vi "Autonomous Independent.vi"() -> ()   [LabVIEW 2015]
doc: "This VI is called when autonomous begins, and will automatically be terminated when autonomous ends. You can carry out timed or sensor driven robot movement independently without needing to return to the caller."
uses:
  <vilib>/Rock Robotics/WPI/SafetyOutput/WPI_SafetyOutputConfigMenu.ctl
  <vilib>/Rock Robotics/WPI/Utilities/WPI_GetSetVariantRefNum.vi
  <vilib>/Rock Robotics/Network Tables/NT Read String.vi
  <vilib>/Rock Robotics/Network Tables/NT Write Numeric Array.vi
  <vilib>/Rock Robotics/Network Tables/NT Read Number.vi
  <vilib>/Rock Robotics/WPI/Ultrasonic/WPI_SonarMB1010AnalogRefNum Registry Get.vi
  navx-mxp/labview/navX Library v2/navX Library v2.lvlib
panel:
  out "Distance":dbl
  out "Numeric 2":dbl
  out "Numeric":dbl
  # "Be sure to right-click and choose Data Operations>>Make Current Value default if you want to save the array values with the VI"
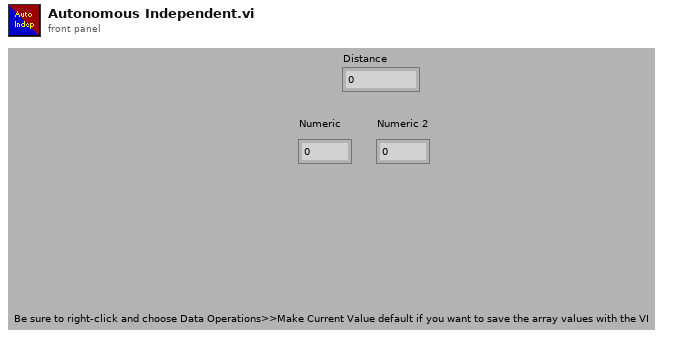
[diagram p1: front panel]
types:
  T1 = typedef "WPI_SafetyOutputConfigMenu.ctl" = enum16{"Enable", "Disable"}
  T2 = typedef "WPI_JoystickDevRef.ctl" = cluster{"Device":T3}
  T3 = typedef "WPI_JoystickDeviceEnum.ctl" = enum16{"USB 0", "USB 1", "USB 2", "USB 3", "USB 4", "USB 5"}
  T4 = typedef "WPI_RobotDriveDevRef.ctl" = cluster{"DevStatus":errorcluster, "Motors[]":T5[], "Square Inputs":bool, "Max Output":dbl}
  T5 = typedef "WPI_MotorControlDeviceRef.ctl" = cluster{"DeviceStatus":errorcluster, "Type":T6, "PWM":cluster{"PWM Channel":T7, "DeadBand":T8}, "CAN":cluster{"Device Number":u8, "Control Mode":T9, "Semaphore":T10, "Max Vout":dbl, "TalonSRX Control Mode":T11}, "Invert":bool}
  T6 = typedef "WPI_MotorControlType.ctl" = enum16{"PWM", "CAN", "CANTalonSRX"}
  T7 = typedef "FPGA_DIOPWMChannel.ctl" = enum8{"PWM 0", "PWM 1", "PWM 2", "PWM 3", "PWM 4", "PWM 5", "PWM 6", "PWM 7", "PWM 8", "PWM 9", "PWM MXP 0", "PWM MXP 1", "PWM MXP 2", "PWM MXP 3", "PWM MXP 4", "PWM MXP 5", "PWM MXP 6", "PWM MXP 7", "PWM MXP 8", "PWM MXP 9", "Invalid"}
  T8 = typedef "WPI_PWMDeadband.ctl" = cluster{"Name":string, "maxPositivePwm":i32, "minPositivePwm":i32, "centerPwm":i32, "maxNegativePwm":i32, "minNegativePwm":i32, "angularRange":u16}
  T9 = typedef "WPI_CANJaguar_ControlMode.ctl" = enum8{"Percent VBus", "Current", "Speed", "Position", "Voltage"}
  T10 = typedef "Semaphore RefNum" = refnum<k1>
  T11 = typedef "WPI_CANTalonSRX_APIControlMode.ctl" = enum8{"Percent VBus", "Speed", "Position", "Slave", "Unchanged / Invalid", "Voltage Compensation", "Current", "Motion Profile"}
  T12 = typedef "navX Library v2.lvlib/Z900_navX_DeviceTypeDef.ctl" = cluster{"Interface":cluster{"Protocol":T13, "Update Rate (4Hz-60Hz)":u8, "navX Open TypeDef":variant}, "Notify Packet":refnum<notifier>, "Loop VI Refnum":refnum<vi>, "Ready to Close Occurrence Refnum":refnum<k4>}
  T13 = typedef "navX Library v2.lvlib/Z900_navX_ProtocolTypeDef.ctl" = enum16{"SERIAL", "I2C", "SPI"}
  T14 = typedef "WPI_EncoderDevRef.ctl" = cluster{"DevStatus":errorcluster, "EncoderIndex":T15, "CounterIndex":T16, "DistancePerCount":dbl, "Decoding Type":T17}
  T15 = typedef "FPGA_EncoderIdx.ctl" = enum8{"Enc 0", "Enc 1", "Enc 2", "Enc 3", "Enc 4", "Enc 5", "Enc 6", "Enc 7", "Invalid"}
  T16 = typedef "FPGA_CounterCtrSystemIndex.ctl" = enum8{"Ctr 0", "Ctr 1", "Ctr 2", "Ctr 3", "Ctr 4", "Ctr 5", "Ctr 6", "Ctr 7", "Invalid"}
  T17 = typedef "WPI_EncoderType.ctl" = enum16{"1x", "2x", "4x"}
  T18 = typedef "WPI_SonarMB1010AnalogDeviceRef.ctl" = cluster{"AIDeviceRef":T19, "Scaling factor (V/in)":dbl, "Average Bits":u8}
  T19 = typedef "WPI_AnalogChannelDevRef.ctl" = cluster{"DevStatus":errorcluster, "Analog Channel":T20}
  T20 = typedef "FPGA_AIChannel.ctl" = enum8{"AI 0", "AI 1", "AI 2", "AI 3", "AI MXP 0", "AI MXP 1", "AI MXP 2", "AI MXP 3", "Invalid"}
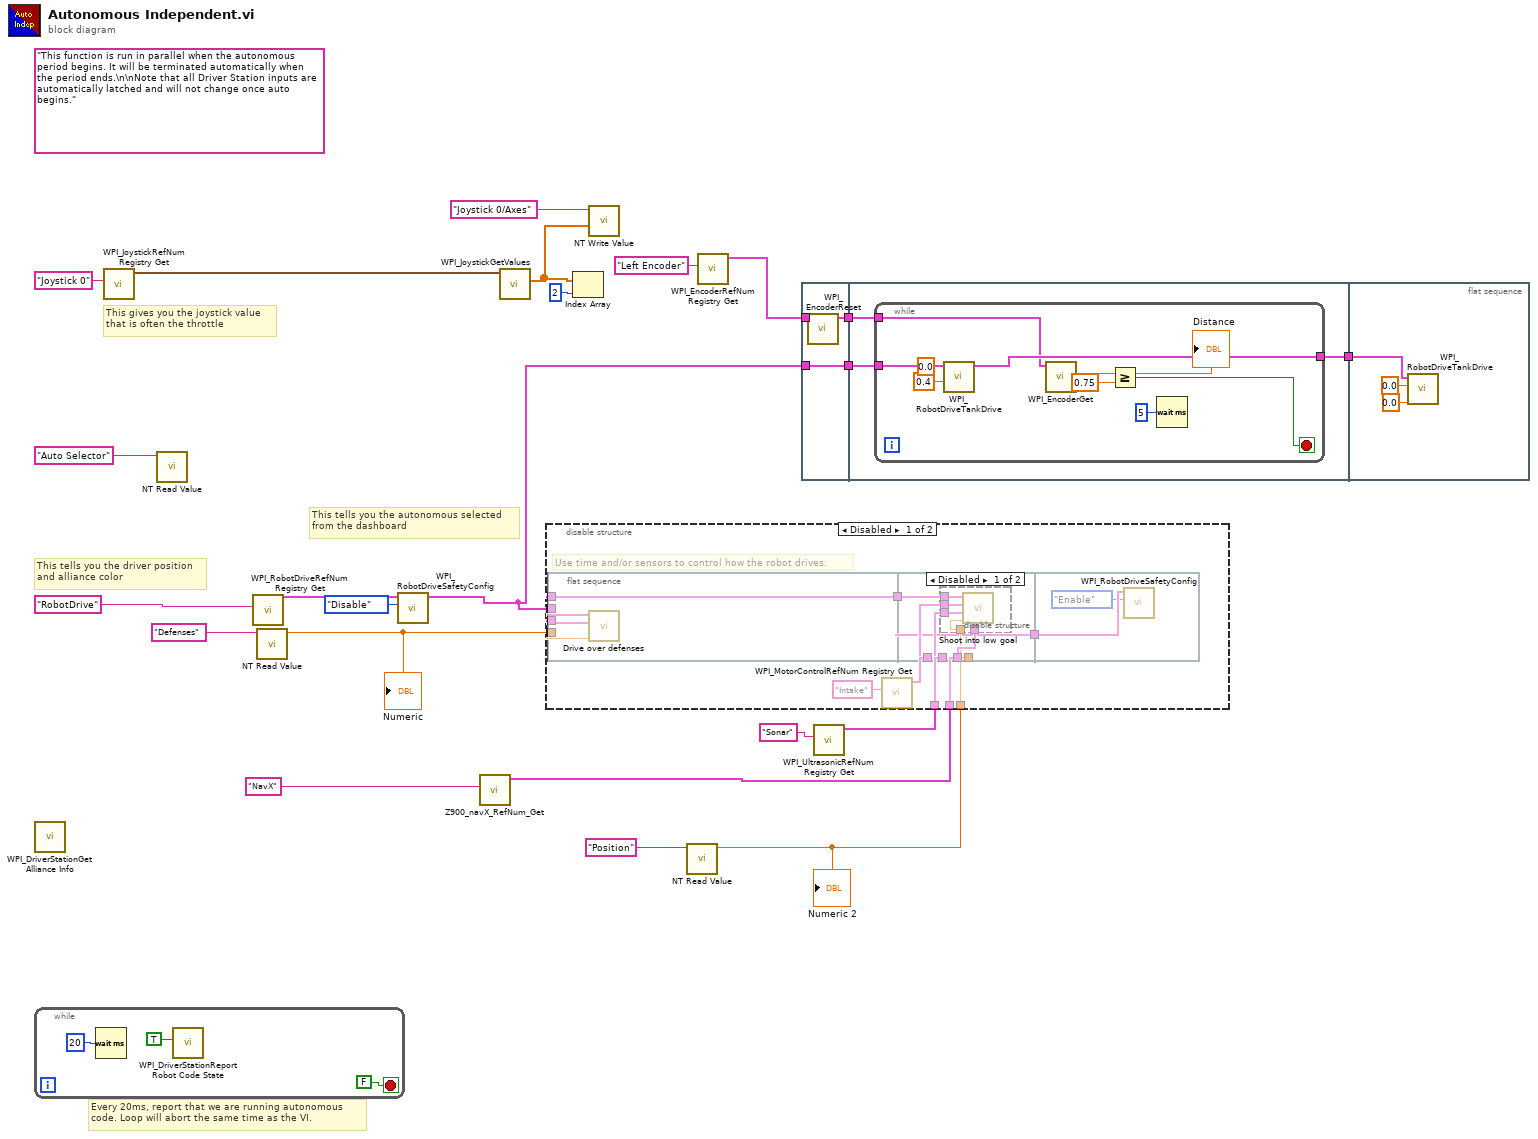
[diagram p0: block diagram]
diagram:
  (unwired) "This function is run in parallel when the autonomous period begins. It will be terminated automatically when the period ends.\n\nNote that all Driver Station inputs are automatically latched and will not change once auto begins."
  # "This tells you the autonomous selected\nfrom the dashboard"
  # "Every 20ms, report that we are running autonomous\ncode. Loop will abort the same time as the VI."
  # "This gives you the joystick value\nthat is often the throttle"
  # "This tells you the driver position\nand alliance color"
  n1 = call <vilib>:"WPI_DriverStationGet Alliance Info.vi"() -> ()  [unwired: 12 out]
  n2 = while {
    stop <- FALSE stop-if-true
    n3 = Wait (ms)(milliseconds to wait=u32 20) -> ()  [unwired: 1 out]
    n4 = call <vilib>:"WPI_DriverStationReport Robot Code State.vi"("Autonomous"=TRUE) -> ()  [unwired: 10 in, 1 out]
  }
  n5 = call <vilib>:"WPI_JoystickRefNum Registry Get.vi"("refnum name"="Joystick 0") -> ("JoystickDevRef"=w22:T2)  [unwired: 1 in, 9 out]
  n6 = call-poly <vilib>:"NT Read Value.vi"("Name"="Auto Selector") -> ()  [unwired: 9 in, 2 out]
  n7 = call <vilib>:"WPI_RobotDriveRefNum Registry Get.vi"("refnum name"="RobotDrive") -> ("RobotDriveDevRef"=w7:T4)  [unwired: 9 in, 1 out]
  n8 = call-poly <vilib>:"NT Read Value.vi"("Name"="Defenses") -> ("Numeric"=w13:dbl)  [unwired: 9 in, 1 out]
  "Numeric" <- w13
  n9 = call <vilib>:"WPI_RobotDriveSafetyConfig.vi"("mode"=WPI_SafetyOutputConfigMenu."Disable", "RobotDriveDevRef"=w7) -> ("RobotDriveDevRef"=w5:T4)  [unwired: 8 in, 1 out]
  n10 = call "Z900_navX_RefNum_Get.vi"("refnum name"="NavX") -> ("navX Device"=w9:T12)  [unwired: 9 in, 1 out]
  n11 = call <vilib>:"WPI_JoystickGetValues.vi"("JoystickDevRef"=w22) -> ("Axes"=w19:dbl[])  [unwired: 6 in, 4 out]
  n12 = Index Array(array=w19, index=2) -> ()  [unwired: 1 out]
  n13 = call-poly <vilib>:"NT Write Value.vi"("Numeric Array"=w19, "Name"="Joystick 0/Axes") -> ()  [unwired: 9 in, 1 out]
  n14 = call-poly <vilib>:"NT Read Value.vi"("Name"="Position") -> ("Numeric"=w8:dbl)  [unwired: 9 in, 1 out]
  "Numeric 2" <- w8
  n15 = call <vilib>:"WPI_EncoderRefNum Registry Get.vi"("refnum name"="Left Encoder") -> ("EncoderDevRef"=w2:T14)  [unwired: 9 in, 1 out]
  n16 = flat-sequence {
    tunnel: w5 -> [w29]
    tunnel: [w29] -> w3
    tunnel: w2 -> [w28]
    tunnel: [w27] -> w1
    tunnel: [w31] -> w4
    tunnel: w3 -> [w32]
    tunnel: w1 -> [w30]
    tunnel: w4 -> [w42]
    frame #0 {
      n17 = call <vilib>:"WPI_EncoderReset.vi"("EncoderDevRef"=w28) -> ("EncoderDevRef"=w27:T14)  [unwired: 9 in, 1 out]
    }
    frame #1 {
      n18 = while {
        tunnel: w32 -> [w41]
        tunnel: [w34] -> w31
        tunnel: w30 -> [w33]
        stop <- w36 stop-if-true
        n19 = call <vilib>:"WPI_RobotDriveTankDrive.vi"("Right axis value"=0.4, "Left axis value"=0.0, "RobotDriveDevRef"=w41) -> ("RobotDriveDevRef"=w34:T4)  [unwired: 6 in, 2 out]
        n20 = call <vilib>:"WPI_EncoderGet.vi"("EncoderDevRef"=w33) -> ("Distance"=w38:dbl)  [unwired: 5 in, 5 out]
        "Distance" <- w38
        n21 = Greater Or Equal?(x=w38, y=0.75) -> (x >= y?=w36:bool)
        n22 = Wait (ms)(milliseconds to wait=u32 5) -> ()  [unwired: 1 out]
      }
    }
    frame #2 {
      n23 = call <vilib>:"WPI_RobotDriveTankDrive.vi"("Right axis value"=0.0, "Left axis value"=0.0, "RobotDriveDevRef"=w42) -> ()  [unwired: 6 in, 3 out]
    }
  }
  n24 = call-poly <vilib>:"WPI_UltrasonicRefNum Registry Get.vi"("refnum name"="Sonar") -> ("SonarMB1010AnalogDevRef"=w10:T18)  [unwired: 9 in, 1 out]
  n25 = disable-structure shown="Disabled" {
    disable-tunnel: w13 -> [w51 _]
    disable-tunnel: w10 -> [w48 _]
    disable-tunnel: w9 -> [w47 _]
    disable-tunnel: w8 -> [w46 _]
    disable-tunnel: w5 -> [w45 _]
    frame Disabled {
      # "Use time and/or sensors to control how the robot drives."
      n26 = flat-sequence {
        tunnel: w47 -> [w57]
        tunnel: w45 -> [w56]
        tunnel: w51 -> [w55]
        tunnel: [w54] -> w53
        tunnel: w45 -> [w54]
        tunnel: w50 -> [w62]
        tunnel: w48 -> [w61]
        tunnel: w47 -> [w60]
        tunnel: w53 -> [w58]
        tunnel: w46 -> [w59]
        tunnel: [w58] -> w52
        tunnel: w52 -> [w69]
        frame #0 {
          n27 = call "Drive over defenses.vi"("Type of Defense"=w55, "navX Device"=w57, "RobotDriveDevRef"=w56) -> ()  [unwired: 9 in]
        }
        frame #1 {
          n28 = disable-structure shown="Disabled" {
            disable-tunnel: w62 -> [w67 _]
            disable-tunnel: w61 -> [w66 _]
            disable-tunnel: w60 -> [w65 _]
            disable-tunnel: w59 -> [w64 _]
            disable-tunnel: w58 -> [w63 _]
            frame Disabled {
              n29 = call "Shoot into low goal.vi"("navX Device"=w65, "Enum"=w64, "SonarMB1010AnalogDevRef"=w66, "MotorControlDevRef"=w67, "RobotDriveDevRef"=w63) -> ()  [unwired: 7 in]
            }
            frame Enabled {
            }
          }
        }
        frame #2 {
          n30 = call <vilib>:"WPI_RobotDriveSafetyConfig.vi"("mode"=WPI_SafetyOutputConfigMenu."Enable", "RobotDriveDevRef"=w69) -> ()  [unwired: 8 in, 2 out]
        }
      }
      n31 = call <vilib>:"WPI_MotorControlRefNum Registry Get.vi"("refnum name"="Intake") -> ("MotorControlDevRef"=w50:T5)  [unwired: 9 in, 1 out]
    }
    frame Enabled {
    }
  }
